vi "Publisher.vi"() -> ()   [LabVIEW 2015]
uses:
  <vilib>/Distrio/LabbitMQ/Connection/Connection.lvclass
  <vilib>/Distrio/LabbitMQ/Connection/connection_parameters_cluster.ctl
  <vilib>/Distrio/LabbitMQ/Channel/exchange_type_enum.ctl
  <vilib>/Distrio/LabbitMQ/Exchange/Exchange.lvclass
  <vilib>/Distrio/LabbitMQ/Channel/Channel.lvclass
panel:
  in  "buttonStop":bool
  in  "Message":string="Hello world!"
  in  "buttonSend":bool
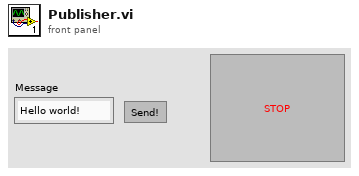
[diagram p1: front panel]
types:
  T1 = typedef "Channel.lvclass/exchange_type_enum.ctl" = enum16{"direct", "topic", "fanout", "headers"}
  T2 = typedef "Connection.lvclass/connection_parameters_cluster.ctl" = cluster{"host name":string, "port":i32, "user name":string, "password":string, "virtual host":string}
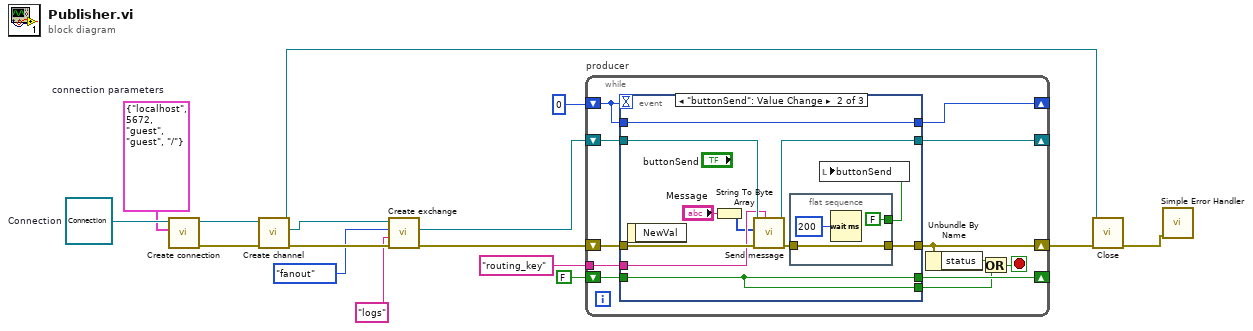
[diagram p0: block diagram]
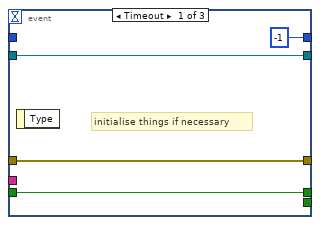
[diagram p2: hidden frame]
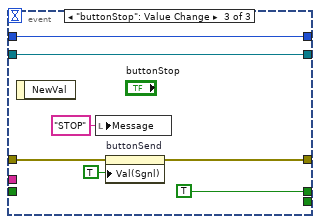
[diagram p3: hidden frame]
diagram:
  w4 = T2 {"host name"="localhost", "port"=5672, "user name"="guest", "password"="guest", "virtual host"="/"}  # connection parameters
  w14 = refnum<class "Connection.lvclass"> refnum  # Connection
  n1 = call <vilib>:"Create connection.vi"("connection parameters"=w4, "Connection in"=w14) -> ("error out"=w10:errorcluster, "Connection out"=w9:refnum<class "Connection.lvclass">)  [unwired: 8 in]
  n2 = call <vilib>:"Create channel.vi"("error in (no error)"=w10, "Connection in"=w9) -> ("error out"=w7:errorcluster, "channel"=w8:refnum<class "Channel.lvclass">, "Connection out"=w12:refnum<class "Connection.lvclass">)  [unwired: 7 in]
  n3 = call <vilib>:"Create exchange.vi"("error in (no error)"=w7, "exchange name"="logs", "exchange type"=exchange_type_enum."fanout" ("binding"), "Channel in"=w8) -> ("error out"=w6:errorcluster, "Exchange.lvclass"=w5:refnum<class "Exchange.lvclass">)  [unwired: 5 in, 1 out]
  n4 = while "producer" {
    shift-right: [w26] -> w11
    shift-left: w6 -> [w27]
    shift-right: [w25] -> _
    shift-left: w5 -> [w28]
    shift-right: [w18] -> _
    shift-left: FALSE -> [w22]
    tunnel: "routing_key" -> [w21]
    shift-right: [w19] -> _
    shift-left: 0 -> [w20]
    stop <- w23 stop-if-true
    n5 = event shown="[1] \"buttonSend\": Value Change" {
      selector: _ -> [_ _ _]
      dyn-events: _ -> [_ _ _]
      timeout: w20 -> [_ _ _]
      tunnel: w28 -> [w32 w38 w53]
      tunnel: w27 -> [w31 w40 w51]
      tunnel: [w31 w34 w50] -> w26
      tunnel: [w32 w39 w53] -> w25
      tunnel: w22 -> [w30 w41 _]
      tunnel: [w30 w41 TRUE] -> w18
      tunnel: w21 -> [_ w37 _]
      tunnel: w20 -> [_ w42 w47]
      tunnel: [-1 w42 w47] -> w19
      tunnel: [_ w41 _] -> w17
      event Timeout {
        # "initialise things if necessary"
        n6 = event-data() -> ()  [unwired: 1 in, 1 out]
      }
      event "buttonSend": Value Change {
        n7 = event-data() -> ()  [unwired: 1 in, 1 out]
        n8 = String To Byte Array(string="Message") -> (unsigned byte array=w36:u8[])
        n9 = call <vilib>:"Send message.vi"("routing key"=w37, "error in (no error)"=w40, "body"=w36, "Exchange in"=w38) -> ("error out"=w35:errorcluster, "Exchange out"=w39:refnum<class "Exchange.lvclass">)  [unwired: 6 in]
        n10 = flat-sequence {
          tunnel: w35 -> [w45]
          tunnel: [w45] -> w34
          tunnel: [FALSE ("buttonSend")] -> w33
          frame #0 {
            n11 = Wait (ms)(milliseconds to wait=u32 200) -> ()  [unwired: 1 out]
          }
        }
        n12 = local write "buttonSend"(w33) -> ()
      }
      event "buttonStop": Value Change {
        n13 = event-data() -> ()  [unwired: 1 in, 1 out]
        n14 = local write "Message"("STOP" ("Message")) -> ()
        n15 = property on="buttonSend" class="Bool (strict)"(error in=w51, "Val(Sgnl)"=TRUE ("Value (Signaling)")) -> (error out=w50:errorcluster)  [unwired: 1 in, 1 out]
      }
    }
    n16 = Unbundle By Name(w26) -> ("status"=w24:bool)
    n17 = Or(x=w24, y=w17) -> (x .or. y?=w23:bool)
  }
  n18 = call <vilib>:"Close.vi"("error in (no error)"=w11, "Connection in"=w12) -> ("error out"=w1:errorcluster)  [unwired: 8 in, 1 out]
  n19 = call <vilib>:"Simple Error Handler.vi"("error in (no error)"=w1) -> ()  [unwired: 4 in, 5 out]
